vi "encode_test_FPGA.vi"() -> ()   [LabVIEW 2014]
uses:
  <vilib>/Platform/TimedLoop/XDataNode/timing_clust.ctl
  <vilib>/Platform/TimedLoop/XDataNode/nitl_modes.ctl
  <vilib>/Platform/TimedLoop/XDataNode/wakeup.ctl
  <vilib>/rvi/Emulation/niFpgaGetClockAttributes.vi
  <vilib>/rvi/Emulation/niFpgaSctlEmulationGetInTimedLoop.vi
  <vilib>/rvi/Emulation/niFpgaEmulationReportErrorSimple.vi
  <vilib>/rvi/eio/common/nirviEmuTemplateMethod_errors.vi
  <vilib>/rvi/DataTransferAndStorage/Container/Common/niFpgaContainerExecOnDevCompGetState.vi
  <vilib>/rvi/Emulation/niFpgaEmulationIsFPGAContextNoSignature.vi
  <vilib>/rvi/errors/niFpgaSetErrorForExecOnDevCompSimple.vi
  <vilib>/rvi/eio/common/nirviEmuReportErrorAndStop.vi
  <vilib>/rvi/DataTransferAndStorage/Container/Common/niFpgaContainerGetUniqueNameForEmu.vi
  <vilib>/rvi/FIFO/Fifo_Resource/nirvififoEmulationSetSize.vi
  <vilib>/rvi/FIFO/Fifo_Resource/nirviFifoEmulationQueueMgr.vi
  <instcachedir>/0/nirviFifoEmulationQueueMgr_E5CAEC123FF24DC58D834DCA3CDAA9B5.lvgen/nirviFifoEmulationQueueMgr_E5CAEC123FF24DC58D834DCA3CDAA9B5_013.vi
  <vilib>/rvi/FIFO/Fifo_Resource/nirvififoEmulationDetermineInputValidOut.vi
  <vilib>/rvi/FIFO/Fifo_Resource/nirvififoEmulationCreateLock.vi
  <vilib>/rvi/Emulation/niFpgaProcessEmulError.vi
  <vilib>/rvi/FIFO/Fifo_Resource/nirvififoEmulationObtainLock.vi
  <vilib>/rvi/FIFO/Fifo_Resource/nirvififoEmulationReleaseLock.vi
  <vilib>/rvi/occurrence/nirviWaitOnOccurrenceBase.vi
  <vilib>/rvi/errors/nirviReportUnexpectedCaseInternalError.vi
  <vilib>/rvi/errors/nirviReportUnexpectedCaseInternalError (U32).vi
  <vilib>/rvi/interface/RandomDataEmulation/niFpgaRandomDataHandleErrors.vi
  <vilib>/rvi/Emulation/niFpgaCriticalErrorInLSC.vi
  <vilib>/eio/EIONode/EIONode.xnode
  <vilib>/rvi/DataTransferAndStorage/Container/XNode/niFpgaContainer.xnode
  <vilib>/rvi/FIFO/Fifo_Resource/niFpgaFifoEmulationRefIn.vi
  <vilib>/Platform/TimedLoop/XDataNode/XDataNode.xnode
  <vilib>/Platform/TimedLoop/XDataNode/XDNodeRunTimeDep.lvlib
  <instrlib>/_niInstr/Basic Elements/v1/FPGA/niInstr Basic Elements v1 FPGA.lvlib
panel:
  out "TRIG0":bool
  in  "manual_data_trig":bool
  in  "reset_data_trig":bool
  out "data_trig":bool
  out "TRIG1":bool
  in  "manual_config_trig":bool
  in  "reset_config_trig":bool
  out "config_trig":bool
  in  "block_trigs":bool
  in  "wait (usec)":u32 caption="Count(uSec)"
  in  "loop timer (usec)":u32=2
  out "loop time":fxp<+,32,32> format="%.39g"
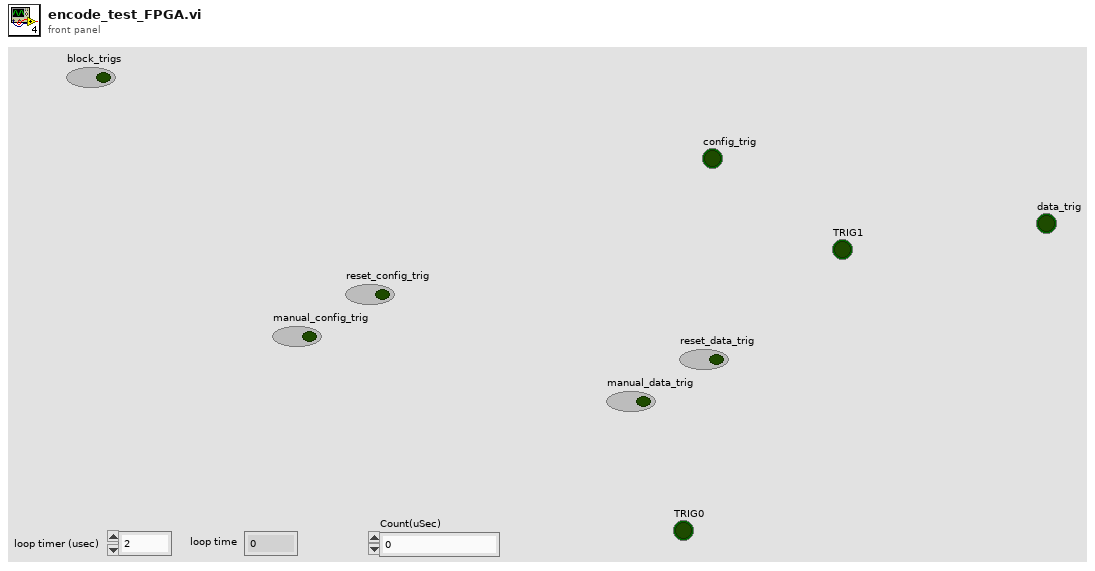
[diagram p1: front panel]
types:
  T1 = typedef "XDNodeRunTimeDep.lvlib/timing_clust.ctl" = cluster{"Expected End [f-1]":u64, "Actual End [f-1]":u64, "Finished Late? [f-1]":bool, "Expected End [i-1]":u64, "Actual End [i-1]":u64, "Finished Late? [i-1]":bool, "Expected Start [i]":u64, "Actual Start [i]":u64, "Expected Start [f]":u64, "Actual Start [f]":u64, "Source Name":string, "Structure Name":string, "Period":i64, "Deadline":i64, "Offset":i64, "Start":i64, "Priority":i32, "Timeout":i32, "Mode":T2, "Wakeup Reason":T3, "Error":errorcluster, "Source Type":string, "Secondary Source Type":string, "Global End Time":u64, "Global Start Time":u64, "Frame Duration":u64, "Iteration Duration":u64, "Assigned CPU":i32, "I/O Scan Engine Mode":u32}
  T2 = typedef "XDNodeRunTimeDep.lvlib/nitl_modes.ctl" = enum32{"No Change", "Process missed periods, maintain original phase", "Discard missed periods, maintain original phase", "Process missed periods, ignore original phase", "Discard missed periods, ignore original phase"}
  T3 = typedef "XDNodeRunTimeDep.lvlib/wakeup.ctl" = enum32{"Normal", "Aborted", "Asynchronous wakeup", "Timing source error", "Timed loop error", "Timeout"}
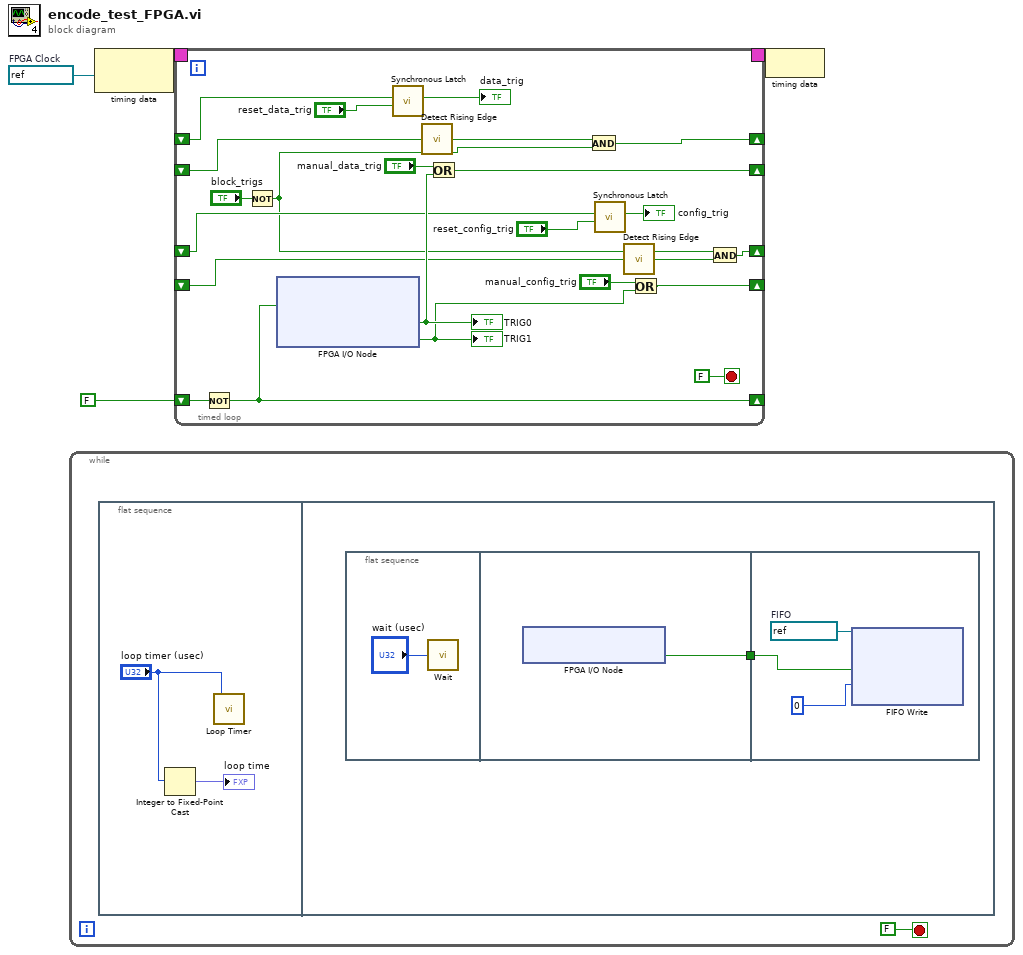
[diagram p0: block diagram]
diagram:
  w2 = refnum<k21> "20MHz"  # FPGA Clock
  n1 = while {
    stop <- FALSE stop-if-true
    n2 = flat-sequence {
      frame #0 {
        n3 = Integer to Fixed-Point Cast(integer="loop timer (usec)") -> (fixed-point=→"loop time":fxp<+,32,32>)  [unwired: 1 in]
        n4 = call "Loop Timer"("Count(uSec)"="loop timer (usec)") -> ()  [unwired: 1 out]
      }
      frame #1 {
        n5 = flat-sequence {
          tunnel: [w10] -> w8
          tunnel: w8 -> [w11]
          frame #0 {
            n6 = call "Wait"("Count(uSec)"="wait (usec)") -> ()  [unwired: 1 out]
          }
          frame #1 {
            n7 = xnode "FPGA I/O Node"() -> ("Connector1/DIO23"=w10:bool)  [unwired: 1 in, 1 out]
          }
          frame #2 {
            w12 = refnum<k21> "encode"  # FIFO
            n8 = xnode ("FIFO Write")("Element"=w11, "Timeout"=0, "FIFO In"=w12) -> ()  [unwired: 2 out]
          }
        }
      }
    }
  }
  n9 = node-c288(w2) -> (w4:T1)
  n10 = timed-loop {
    timing: w4 -> [_]
    timing-out: [_] -> w3
    shift-right: [w34] -> _
    shift-left: FALSE -> [w35]
    shift-right: [w31] -> _
    shift-left: _ -> [w30]
    shift-right: [w18] -> _
    shift-left: _ -> [w19]
    shift-right: [w23] -> _
    shift-left: _ -> [w22]
    shift-right: [w17] -> _
    shift-left: _ -> [w21]
    stop <- FALSE stop-if-true
    n11 = Not(x=w35) -> (.not. x?=w34:bool)
    n12 = Not(x="block_trigs") -> (.not. x?=w14:bool)
    n13 = xnode "FPGA I/O Node"("Connector1/DIO25"=w34) -> ("PXI_Trig0"=w33:bool, "PXI_Trig1"=w24:bool)  [unwired: 3 in, 3 out]
    "TRIG0" <- w33
    "TRIG1" <- w24
    n14 = call <instrlib>:"Synchronous Latch.vi"("clear"="reset_data_trig", "set"=w19) -> ("out"=→"data_trig":bool)  [unwired: 9 in]
    n15 = call <instrlib>:"Detect Rising Edge.vi"("signal"=w30) -> ("edge detected"=w16:bool)  [unwired: 14 in]
    n16 = Or(x="manual_data_trig", y=w33) -> (x .or. y?=w31:bool)
    n17 = And(x=w16, y=w14) -> (x .and. y?=w18:bool)
    n18 = call <instrlib>:"Synchronous Latch.vi"("clear"="reset_config_trig", "set"=w21) -> ("out"=→"config_trig":bool)  [unwired: 9 in]
    n19 = call <instrlib>:"Detect Rising Edge.vi"("signal"=w22) -> ("edge detected"=w15:bool)  [unwired: 14 in]
    n20 = Or(x="manual_config_trig", y=w24) -> (x .or. y?=w23:bool)
    n21 = And(x=w14, y=w15) -> (x .and. y?=w17:bool)
  }
  n22 = node-c288(w3) -> ()
